vi "Configure Dialog.vi"(8 "error in (no error)":errorcluster, 11 "Clear Arbitrary Sequence [SEQ] Msg in":refnum<class "Clear Arbitrary Sequence [SEQ] Msg.lvclass">) -> (0 "error out":errorcluster, 2 "Ok?":bool, 3 "Clear Arbitrary Sequence [SEQ] Msg out":refnum<class "Clear Arbitrary Sequence [SEQ] Msg.lvclass">)   [LabVIEW 2015, in "CS++Fgen.lvlib" / "Clear Arbitrary Sequence [SEQ] Msg.lvclass"]
uses:
  Clear Arbitrary Sequence [SEQ] Msg.lvclass
  CSPP_Core/Actors/CS++PVMonitor Messages/CS++PVUpdate Msg/CS++PVUpdate Msg.lvclass
panel:
  in  "sequence handle (0)":i32 caption="Sequence handle"
  in  "OK Button":bool
  in  "Cancel Button":bool
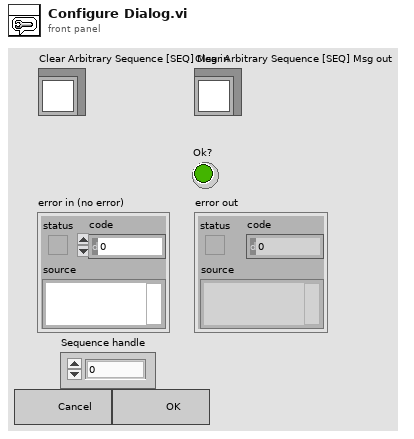
[diagram p1: front panel]
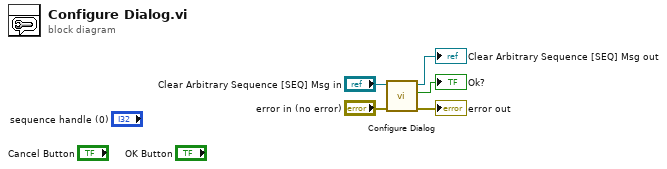
[diagram p0: block diagram]
diagram:
  n1 = call-parent "Configure Dialog.vi"("Error In"="error in (no error)", "Message in"="Clear Arbitrary Sequence [SEQ] Msg in") -> ("Error Out"=→"error out":errorcluster, "OK?"=→"Ok?":bool, "Message out"=→"Clear Arbitrary Sequence [SEQ] Msg out":refnum<class "Clear Arbitrary Sequence [SEQ] Msg.lvclass">)  [unwired: 7 in]
